vi "IMAQdx Acquisition Template (Host)withExtreme.vi"() -> ()   [LabVIEW 2016]
uses:
  <vilib>/userdefined/High Color/IMAQdx.ctl
  <vilib>/vision/driver/IMAQdx.llb/IMAQdx Acquisition Mode.ctl
  <vilib>/vision/driver/IMAQdx.llb/IMAQdx Buffer Number Mode.ctl
  <vilib>/FPGAPlugInAG/roboRIO/niLvFpga_Open_roboRIO.vi
  <vilib>/rvi/interface/common/dynamic/niFpgaDynamicAddResources.vi
  <vilib>/FPGAPlugInAG/Dynamic/niLvFpga_Download_Dynamic.vi
  <vilib>/FPGAPlugInAG/Dynamic/niLvFpga_Run_Dynamic.vi
  <vilib>/visionFPGA/Basics/Configure Image Transfer to Target/IMAQ FPGA Configure Image Transfer to Target U32.vi
  <vilib>/Utility/error.llb/Error Cluster From Error Code.vi
  <vilib>/rvi/errors/niLvFpgaAdjustHostInterfaceError.vi
  <vilib>/visionFPGA/Basics/Image Transfer to Target/IMAQ FPGA Image Transfer to Target U32.vi
  <vilib>/rvi/interface/common/niFpgaWaitOnOcc.vi
  <vilib>/FPGAPlugInAG/Dynamic/niLvFpga_Close_Dynamic.vi
  <vilib>/rvi/interface/nirviOpenFPGA/nirviOpenFPGA.xnode
  FPGA Bitfiles/ImageProcessingw_FPGATarget2_ImageProcessingw_ZcF2hsHpmf8.lvbitx
  <vilib>/rvi/interface/nirviMethod/nirviMethod.xnode
  <vilib>/rvi/interface/nirviReadWriteControl/nirviReadWriteControl.xnode
  <vilib>/rvi/interface/nirviCloseFPGA/nirviCloseFPGA.xnode
  <vilib>/vision/driver/NI_Vision_Acquisition_Software.lvlib
  <resource>/objmgr/imaqdx.rc
  <vilib>/visionFPGA/NI_VDM_FPGA_Basics.lvlib
  <vilib>/rvi/interface/Simulation/niFpgaSimulationCallBeginRW.vi
  <vilib>/rvi/errors/niLvFpgaMergeErrorWithErrorCode.vi
  <vilib>/FPGAPlugInAG/Dynamic/niLvFpga_ReadFifo_Dynamic.vi
  <vilib>/FPGAPlugInAG/Dynamic/niLvFpga_ConfigureFifo_Dynamic.vi
  <vilib>/FPGAPlugInAG/Dynamic/niLvFpga_StartFifo_Dynamic.vi
  NiFpgaLv.dll
panel:
  out "OriImage Err out":errorcluster
  out "Image":T1(plugin-control)
  out "Count":i32
  out "error out 2":errorcluster
  in  "Camera":T2
  out "Error Out":errorcluster
  in  "Stop":bool
  # "Overview: Demonstrates how to acquire an image from a camera using the IMAQdx API, transfer the image to a FPGA target for processing, and retrieve the processed image for display or further processing on the host.\nRequirements:\n- LabVIEW FPGA\n- Vision Acquisition Software\n- Vision Development Module\nInstructions:\n1. Select a Camera\n2. Run the VI."
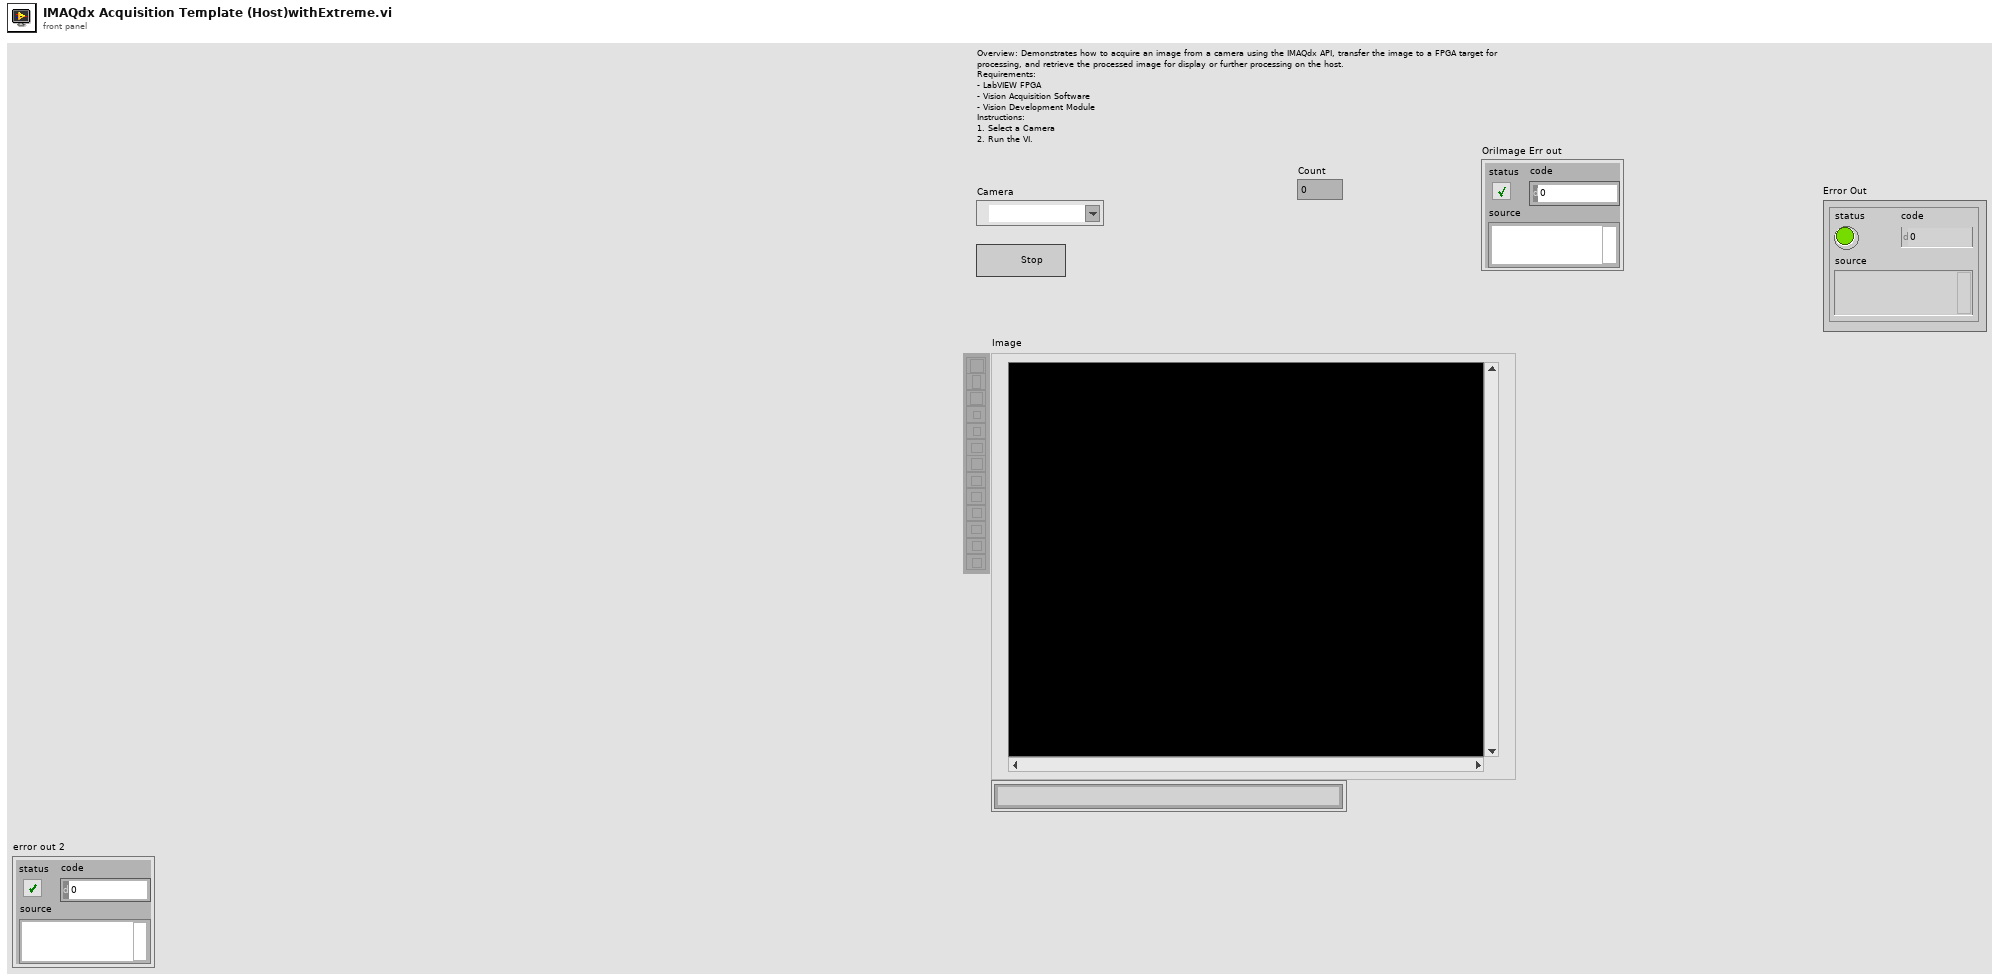
[diagram p1: front panel]
types:
  T1 = typedef "IMAQ Image.ctl" = refnum<image>
  T2 = typedef "IMAQdx.ctl" = refnum<k21>
  T3 = typedef "Image Type" = u32
  T4 = typedef "NI_Vision_Acquisition_Software.lvlib/IMAQdx Acquisition Mode.ctl" = enum32{"One Shot", "Continuous"}
  T5 = typedef "NI_Vision_Acquisition_Software.lvlib/IMAQdx Buffer Number Mode.ctl" = enum32{"Next", "Last", "Buffer Number", "Every", "Last New"}
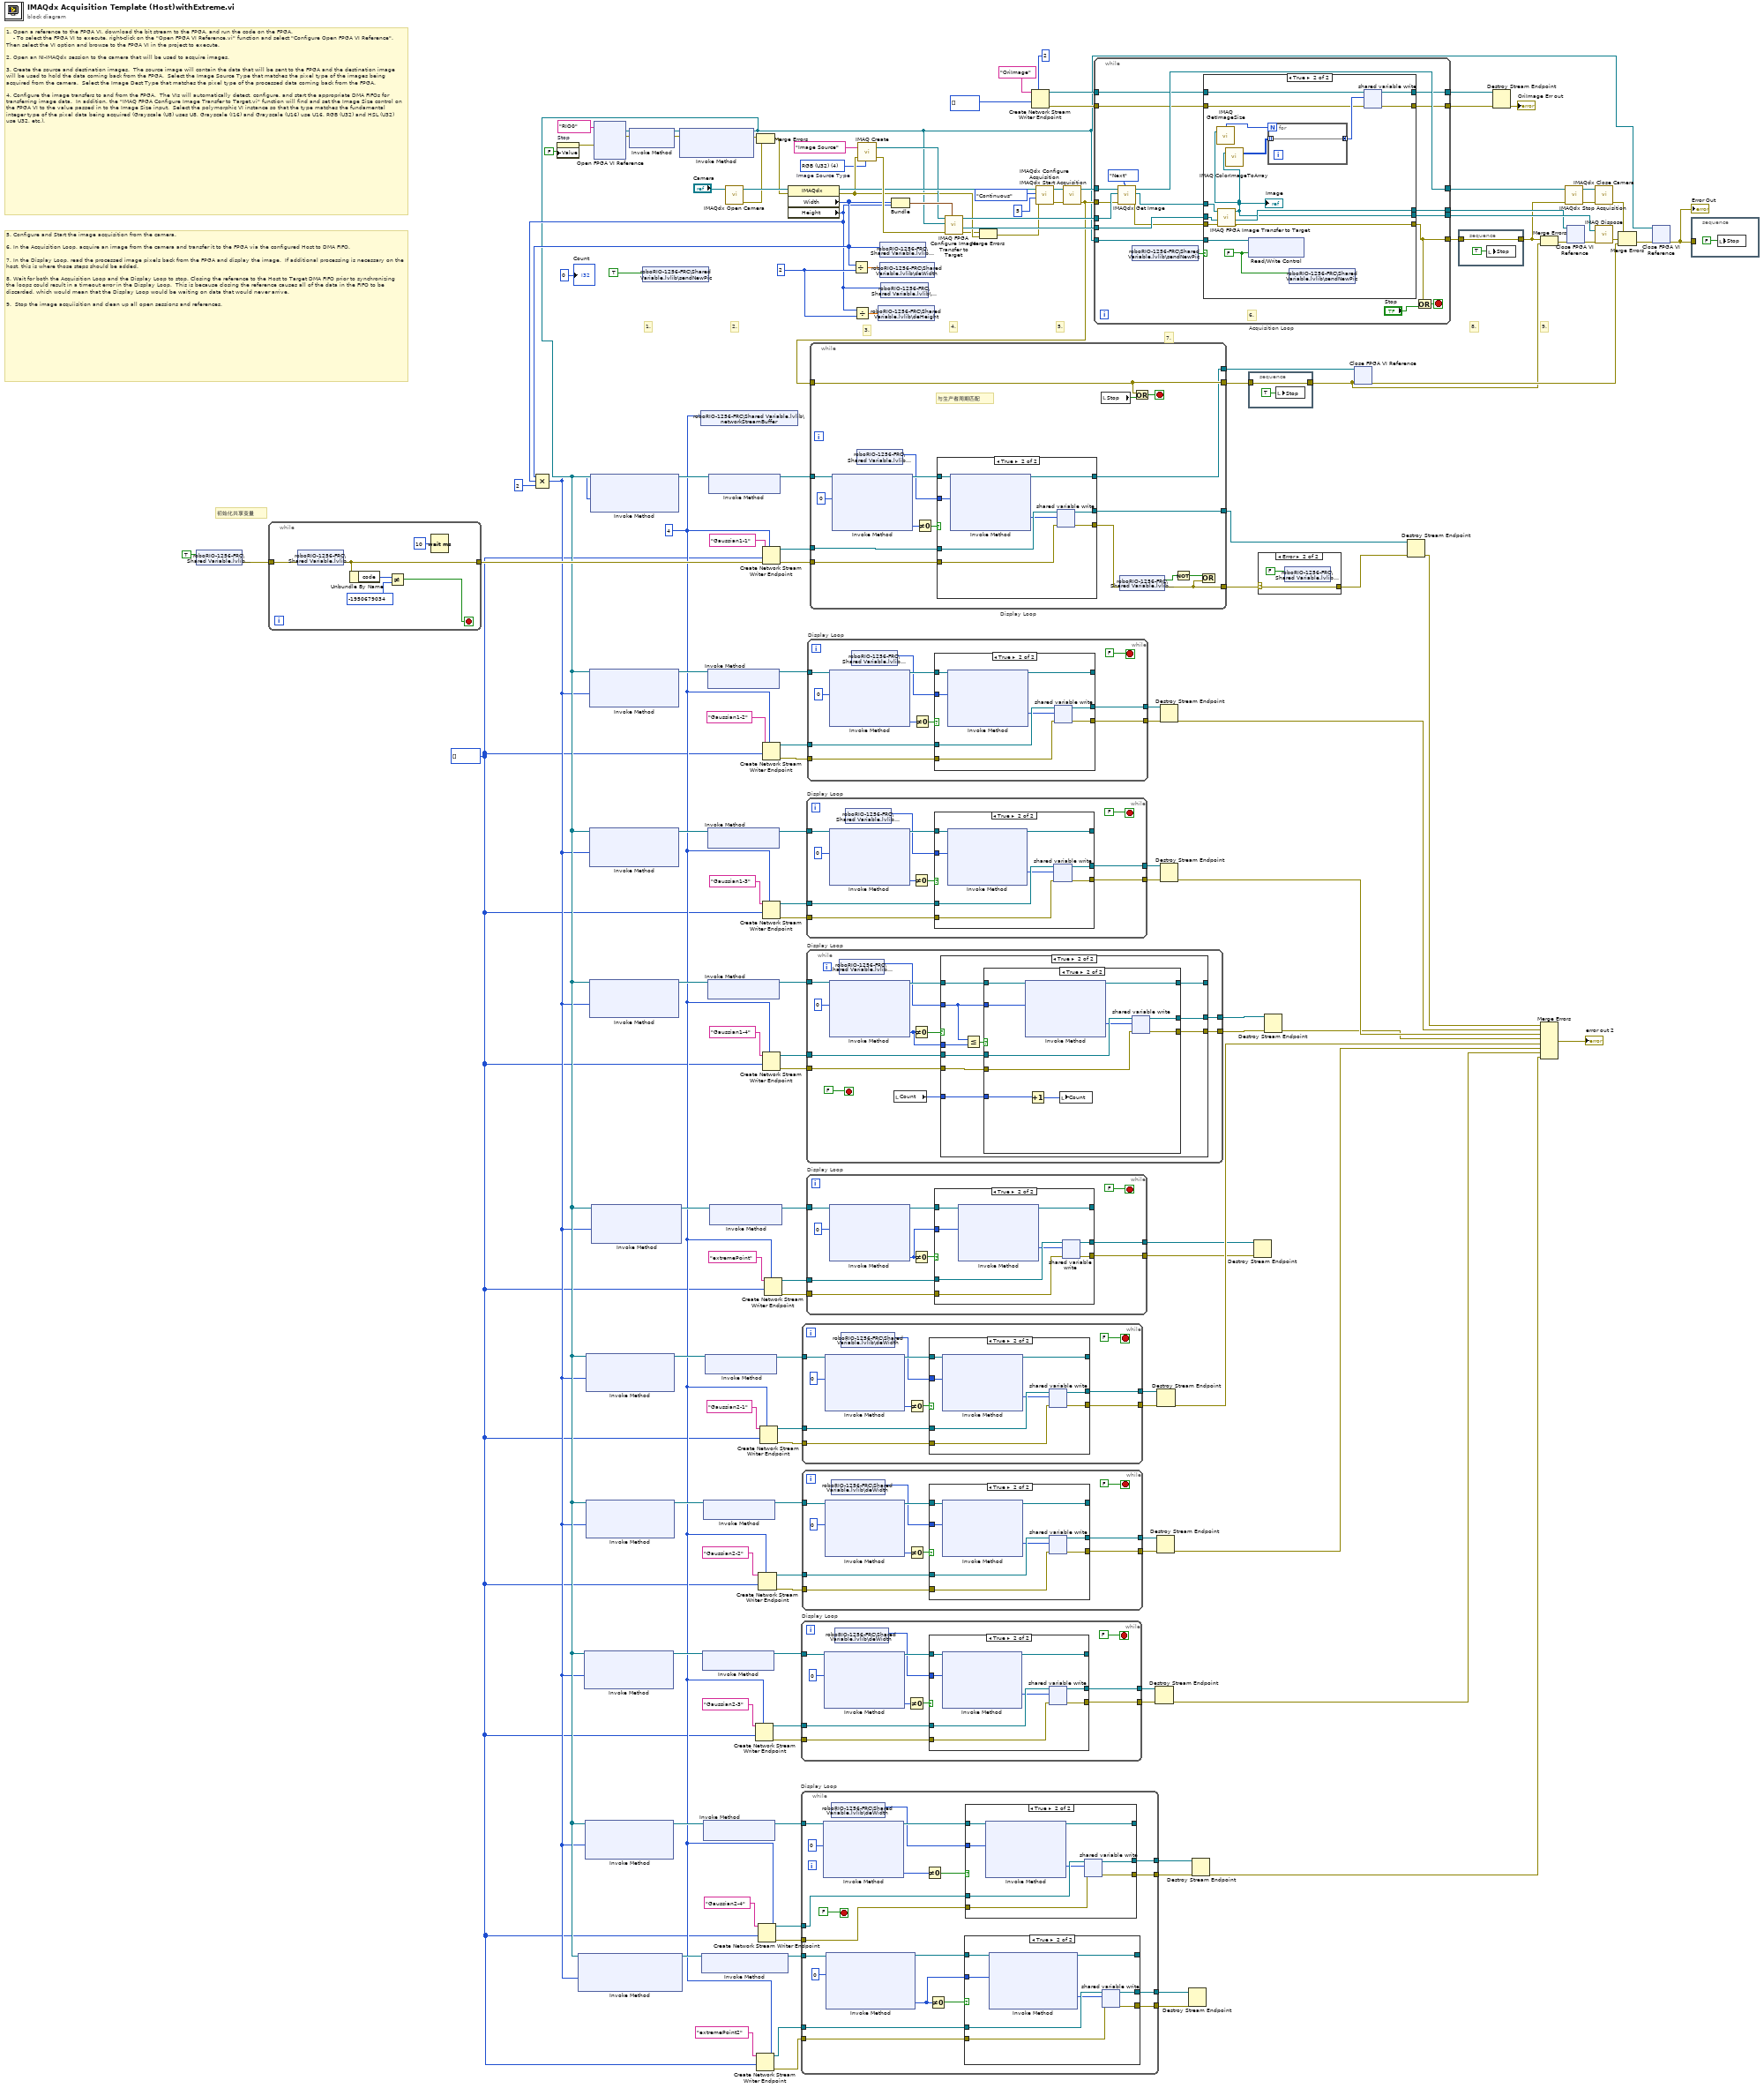
[diagram p0: block diagram]
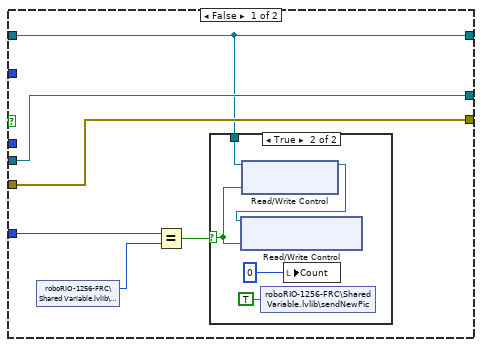
[diagram p6: hidden frame]
diagram:
  w21 = u32 2 ("y")
  w10 = i32[] []
  w12 = 4 ("writer buffer size")
  w112 = T3 4 items=["Grayscale (U8)", "Grayscale (I16)", "Grayscale (SGL)", "Complex (CSG)", "RGB (U32)", "HSL (U32)", "RGB (U64)", "Grayscale (U16)"]  # Image Source Type
  # "初始化共享变量"
  # "5. Configure and Start the image acquisition from the camera.\n\n6. In the Acquisition Loop, acquire an image from the camera and transfer it to the FPGA via the configured Host to DMA FIFO.\n\n7. In the Display Loop, read the processed image pixels back from the FPGA and display the image.  If additional processing is necessary on the host, this is where those steps should be added.\n\n8. Wait for both the Acquisition Loop and the Display Loop to stop. Closing the reference to the Host to Target DMA FIFO prior to synchronizing the loops could result in a timeout error in the Display Loop.  This is because closing the reference causes all of the data in the FIFO to be discarded, which would mean that the Display Loop would be waiting on data that would never arrive.\n\n9.  Stop the image acquiisition and clean up all open sessions and references."
  # "1. Open a reference to the FPGA VI, download the bit stream to the FPGA, and run the code on the FPGA.\n    - To select the FPGA VI to execute, right-click on the \"Open FPGA VI Reference.vi\" function and select \"Configure Open FPGA VI Reference\".  Then select the VI option and browse to the FPGA VI in the project to execute.\n\n2. Open an NI-IMAQdx session to the camera that will be used to acquire images.\n\n3. Create the source and destination images.  The source image will contain the data that will be sent to the FPGA and the destination image will be used to hold the data coming back from the FPGA.  Select the Image Source Type that matches the pixel type of the images being acquired from the camera.  Select the Image Dest Type that matches the pixel type of the processed data coming back from the FPGA.\n\n4. Configure the image transfers to and from the FPGA.  The VIs will automatically detect, configure, and start the appropriate DMA FIFOs for transferring image data.  In addition, the \"IMAQ FPGA Configure Image Transfer to Target.vi\" function will find and set the Image Size control on the FPGA VI to the value passed in to the Image Size input.  Select the polymorphic VI instance so that the type matches the fundamental integer type of the pixel data being acquired (Grayscale (U8) uses U8, Grayscale (I16) and Grayscale (U16) use U16, RGB (U32) and HSL (U32) use U32, etc.)."
  # "9."
  # "8."
  # "7."
  # "6."
  # "5."
  # "4."
  # "3."
  # "2."
  # "1."
  n1 = shared-variable "roboRIO-1256-FRC\\Shared Variable.lvlib\\Active"(TRUE ("Active?")) -> (error out=w98:errorcluster)  [unwired: 1 in]
  n2 = while {
    tunnel: w98 -> [w155]
    tunnel: [w152] -> w97
    stop <- w151 stop-if-true
    n3 = shared-variable "roboRIO-1256-FRC\\Shared Variable.lvlib\\Active"(error in=w155) -> (error out=w152:errorcluster)  [unwired: 1 out]
    n4 = Unbundle By Name(w152) -> ("code"=w154:i32)
    n5 = Not Equal?(x=w154, y=-1950679034) -> (x != y?=w151:bool)
    n6 = Wait (ms)(milliseconds to wait=u32 10) -> ()  [unwired: 1 out]
  }
  n7 = property on="Stop" class="Bool (strict)"("Value"=FALSE ("Stop")) -> (error out=w147:errorcluster)  [unwired: 2 in, 1 out]
  n8 = xnode "Open FPGA VI Reference"("error in"=w147, "resource name"=tag "RIO0") -> ("FPGA VI Reference Out"=w143:refnum<k20>, "error out"=w144:errorcluster)
  n9 = xnode "Invoke Method"("FPGA VI Reference In"=w143, "error in"=w144) -> ("FPGA VI Reference Out"=w146:refnum<k20>, "error out"=w145:errorcluster)
  n10 = shared-variable "roboRIO-1256-FRC\\Shared Variable.lvlib\\sendNewPic"(TRUE) -> ()  [unwired: 1 in, 1 out]
  n11 = xnode "Invoke Method"("FPGA VI Reference In"=w146, "error in"=w145) -> ("FPGA VI Reference Out"=w14:refnum<k20>, "error out"=w132:errorcluster)  [unwired: 1 in]
  n12 = shared-variable "roboRIO-1256-FRC\\Shared Variable.lvlib\\networkStreamBuffer"(w12) -> ()  [unwired: 1 in, 1 out]
  n13 = call <vilib>:"IMAQdx Open Camera.vi"("Session In"="Camera") -> ("error out"=w117:errorcluster, "Session Out"=w118:T2)  [unwired: 9 in]
  n14 = Create Network Stream Writer Endpoint(7:w12, 9:w10, 11:"Gaussian2-3" ("writer name")) -> (0:w34:errorcluster, 3:w33:refnum<k21>)  [unwired: 4 in]
  n15 = Create Network Stream Writer Endpoint(7:w12, 9:w10, 11:"extremePoint2" ("writer name")) -> (0:w8:errorcluster, 3:w9:refnum<k21>)  [unwired: 4 in]
  n16 = Merge Errors(w132, w117) -> (w116:errorcluster)
  n17 = Create Network Stream Writer Endpoint(7:w12, 9:w10, 11:"Gaussian2-4" ("writer name")) -> (0:w59:errorcluster, 3:w60:refnum<k21>)  [unwired: 4 in]
  n18 = Create Network Stream Writer Endpoint(7:w12, 9:w10, 11:"Gaussian2-2" ("writer name")) -> (0:w41:errorcluster, 3:w42:refnum<k21>)  [unwired: 4 in]
  n19 = Create Network Stream Writer Endpoint(7:w12, 9:w10, 11:"Gaussian2-1" ("writer name")) -> (0:w48:errorcluster, 3:w47:refnum<k21>)  [unwired: 4 in]
  n20 = Create Network Stream Writer Endpoint(7:w12, 8:w97, 9:w10, 11:"Gaussian1-1" ("writer name")) -> (0:w93:errorcluster, 3:w92:refnum<k21>)  [unwired: 3 in]
  n21 = Create Network Stream Writer Endpoint(7:w12, 9:w10, 11:"Gaussian1-2" ("writer name")) -> (0:w74:errorcluster, 3:w75:refnum<k21>)  [unwired: 4 in]
  n22 = Create Network Stream Writer Endpoint(7:w12, 9:w10, 11:"Gaussian1-3" ("writer name")) -> (0:w69:errorcluster, 3:w68:refnum<k21>)  [unwired: 4 in]
  n23 = Create Network Stream Writer Endpoint(7:w12, 9:w10, 11:"Gaussian1-4" ("writer name")) -> (0:w53:errorcluster, 3:w54:refnum<k21>)  [unwired: 4 in]
  n24 = Create Network Stream Writer Endpoint(7:w12, 9:w10, 11:"extremePoint" ("writer name")) -> (0:w3:errorcluster, 3:w4:refnum<k21>)  [unwired: 4 in]
  n25 = property class="IMAQdx"(reference=w118, error in=w116) -> (reference out=w125:T2, error out=w113:errorcluster, "Width"=w23:u32, "Height"=w20:u32)
  n26 = Compound Arithmetic op=MULTIPLY(w23, w20, u32 2 ("value")) -> (w13:u32)
  n27 = xnode "Invoke Method"("FPGA VI Reference In"=w14, "Requested Depth"=w13) -> ("FPGA VI Reference Out"=w16:refnum<k20>)  [unwired: 1 in, 2 out]
  n28 = xnode "Invoke Method"("FPGA VI Reference In"=w14, "Requested Depth"=w13) -> ("FPGA VI Reference Out"=w35:refnum<k20>)  [unwired: 1 in, 2 out]
  n29 = xnode "Invoke Method"("FPGA VI Reference In"=w14, "Requested Depth"=w13) -> ("FPGA VI Reference Out"=w58:refnum<k20>)  [unwired: 1 in, 2 out]
  n30 = xnode "Invoke Method"("FPGA VI Reference In"=w14, "Requested Depth"=w13) -> ("FPGA VI Reference Out"=w30:refnum<k20>)  [unwired: 1 in, 2 out]
  n31 = xnode "Invoke Method"("FPGA VI Reference In"=w14, "Requested Depth"=w13) -> ("FPGA VI Reference Out"=w40:refnum<k20>)  [unwired: 1 in, 2 out]
  n32 = xnode "Invoke Method"("FPGA VI Reference In"=w14, "Requested Depth"=w13) -> ("FPGA VI Reference Out"=w73:refnum<k20>)  [unwired: 1 in, 2 out]
  n33 = xnode "Invoke Method"("FPGA VI Reference In"=w14, "Requested Depth"=w13) -> ("FPGA VI Reference Out"=w70:refnum<k20>)  [unwired: 1 in, 2 out]
  n34 = xnode "Invoke Method"("FPGA VI Reference In"=w14, "Requested Depth"=w13) -> ("FPGA VI Reference Out"=w52:refnum<k20>)  [unwired: 1 in, 2 out]
  n35 = xnode "Invoke Method"("FPGA VI Reference In"=w14, "Requested Depth"=w13) -> ("FPGA VI Reference Out"=w102:refnum<k20>)  [unwired: 1 in, 2 out]
  n36 = xnode "Invoke Method"("FPGA VI Reference In"=w14, "Requested Depth"=w13) -> ("FPGA VI Reference Out"=w17:refnum<k20>)  [unwired: 1 in, 2 out]
  n37 = xnode "Invoke Method"("FPGA VI Reference In"=w16) -> ("FPGA VI Reference Out"=w11:refnum<k20>)  [unwired: 1 in, 1 out]
  n38 = xnode "Invoke Method"("FPGA VI Reference In"=w35) -> ("FPGA VI Reference Out"=w36:refnum<k20>)  [unwired: 1 in, 1 out]
  n39 = xnode "Invoke Method"("FPGA VI Reference In"=w58) -> ("FPGA VI Reference Out"=w57:refnum<k20>)  [unwired: 1 in, 1 out]
  n40 = xnode "Invoke Method"("FPGA VI Reference In"=w40) -> ("FPGA VI Reference Out"=w39:refnum<k20>)  [unwired: 1 in, 1 out]
  n41 = xnode "Invoke Method"("FPGA VI Reference In"=w30) -> ("FPGA VI Reference Out"=w29:refnum<k20>)  [unwired: 1 in, 1 out]
  n42 = xnode "Invoke Method"("FPGA VI Reference In"=w73) -> ("FPGA VI Reference Out"=w72:refnum<k20>)  [unwired: 1 in, 1 out]
  n43 = xnode "Invoke Method"("FPGA VI Reference In"=w70) -> ("FPGA VI Reference Out"=w71:refnum<k20>)  [unwired: 1 in, 1 out]
  n44 = xnode "Invoke Method"("FPGA VI Reference In"=w52) -> ("FPGA VI Reference Out"=w51:refnum<k20>)  [unwired: 1 in, 1 out]
  n45 = xnode "Invoke Method"("FPGA VI Reference In"=w102) -> ("FPGA VI Reference Out"=w101:refnum<k20>)  [unwired: 1 in, 1 out]
  n46 = xnode "Invoke Method"("FPGA VI Reference In"=w17) -> ("FPGA VI Reference Out"=w5:refnum<k20>)  [unwired: 1 in, 1 out]
  n47 = while "Display Loop" {
    tunnel: [w175] -> w63
    tunnel: w59 -> [w174]
    tunnel: w60 -> [w173]
    tunnel: [w168] -> w62
    tunnel: w57 -> [w167]
    tunnel: w11 -> [w161]
    tunnel: w9 -> [w160]
    tunnel: w8 -> [w159]
    tunnel: [w158] -> w7
    tunnel: [w157] -> w6
    stop <- FALSE stop-if-true
    n48 = xnode "Invoke Method"("FPGA VI Reference In"=w167, "Number of Elements"=u32 0) -> ("FPGA VI Reference Out"=w170:refnum<k20>, "Elements Remaining"=w165:u32)  [unwired: 2 in, 2 out]
    n49 = xnode "Invoke Method"("FPGA VI Reference In"=w161, "Number of Elements"=u32 0) -> ("FPGA VI Reference Out"=w164:refnum<k20>, "Elements Remaining"=w156:u32)  [unwired: 2 in, 2 out]
    n50 = shared-variable "roboRIO-1256-FRC\\Shared Variable.lvlib\\deWidth"() -> (w166:u16)  [unwired: 1 in, 1 out]
    n51 = Not Equal To 0?(x=w165) -> (x != 0?=w172:bool)
    n52 = Not Equal To 0?(x=w156) -> (x != 0?=w162:bool)
    n53 = case shown="True" w162 {
      tunnel: w164 -> [w176 w186]
      tunnel: [w178 w185] -> w158
      tunnel: w159 -> [w177 w184]
      tunnel: w160 -> [w178 w183]
      tunnel: [w177 w182] -> w157
      tunnel: [w176 w181] -> _
      tunnel: w156 -> [_ w179]
      frame False {
      }
      frame True {
        n54 = xnode "Invoke Method"("FPGA VI Reference In"=w186, "Number of Elements"=w179) -> ("FPGA VI Reference Out"=w181:refnum<k20>, "Data"=w180:u16[])  [unwired: 2 in, 2 out]
        n55 = shared-variable-write(w183, w184, w180) -> (w185:refnum<k21>, w182:errorcluster)  [unwired: 1 in, 1 out]
      }
    }
    n56 = case shown="True" w172 {
      tunnel: w170 -> [w187 w197]
      tunnel: [w189 w196] -> w175
      tunnel: w174 -> [w188 w195]
      tunnel: w173 -> [w189 w194]
      tunnel: [w188 w193] -> w168
      tunnel: [w187 w192] -> _
      tunnel: w166 -> [_ w191]
      frame False {
      }
      frame True {
        n57 = xnode "Invoke Method"("FPGA VI Reference In"=w197, "Number of Elements"=w191) -> ("FPGA VI Reference Out"=w192:refnum<k20>, "Data"=w190:u8[])  [unwired: 2 in, 2 out]
        n58 = shared-variable-write(w194, w195, w190) -> (w196:refnum<k21>, w193:errorcluster)  [unwired: 1 in, 1 out]
      }
    }
  }
  n59 = while "Display Loop" {
    tunnel: [w208] -> w31
    tunnel: w34 -> [w207]
    tunnel: w33 -> [w206]
    tunnel: [w200] -> w32
    tunnel: w36 -> [w199]
    stop <- FALSE stop-if-true
    (unwired) u32 640 ("Number of Elements")
    n60 = xnode "Invoke Method"("FPGA VI Reference In"=w199, "Number of Elements"=u32 0) -> ("FPGA VI Reference Out"=w202:refnum<k20>, "Elements Remaining"=w203:u32)  [unwired: 2 in, 2 out]
    n61 = shared-variable "roboRIO-1256-FRC\\Shared Variable.lvlib\\deWidth"() -> (w198:u16)  [unwired: 1 in, 1 out]
    n62 = Not Equal To 0?(x=w203) -> (x != 0?=w205:bool)
    n63 = case shown="True" w205 {
      tunnel: w202 -> [w209 w219]
      tunnel: [w211 w218] -> w208
      tunnel: w207 -> [w210 w217]
      tunnel: w206 -> [w211 w216]
      tunnel: [w210 w215] -> w200
      tunnel: [w209 w213] -> _
      tunnel: w198 -> [_ w212]
      frame False {
      }
      frame True {
        n64 = xnode "Invoke Method"("FPGA VI Reference In"=w219, "Number of Elements"=w212) -> ("FPGA VI Reference Out"=w213:refnum<k20>, "Data"=w214:u8[])  [unwired: 2 in, 2 out]
        n65 = shared-variable-write(w216, w217, w214) -> (w218:refnum<k21>, w215:errorcluster)  [unwired: 1 in, 1 out]
      }
    }
  }
  n66 = while "Display Loop" {
    tunnel: [w230] -> w45
    tunnel: w48 -> [w229]
    tunnel: w47 -> [w228]
    tunnel: [w222] -> w46
    tunnel: w29 -> [w221]
    stop <- FALSE stop-if-true
    (unwired) u32 640 ("Number of Elements")
    n67 = xnode "Invoke Method"("FPGA VI Reference In"=w221, "Number of Elements"=u32 0) -> ("FPGA VI Reference Out"=w224:refnum<k20>, "Elements Remaining"=w225:u32)  [unwired: 2 in, 2 out]
    n68 = shared-variable "roboRIO-1256-FRC\\Shared Variable.lvlib\\deWidth"() -> (w220:u16)  [unwired: 1 in, 1 out]
    n69 = Not Equal To 0?(x=w225) -> (x != 0?=w227:bool)
    n70 = case shown="True" w227 {
      tunnel: w224 -> [w231 w241]
      tunnel: [w233 w240] -> w230
      tunnel: w229 -> [w232 w239]
      tunnel: w228 -> [w233 w238]
      tunnel: [w232 w237] -> w222
      tunnel: [w231 w235] -> _
      tunnel: w220 -> [_ w234]
      frame False {
      }
      frame True {
        n71 = xnode "Invoke Method"("FPGA VI Reference In"=w241, "Number of Elements"=w234) -> ("FPGA VI Reference Out"=w235:refnum<k20>, "Data"=w236:u8[])  [unwired: 2 in, 2 out]
        n72 = shared-variable-write(w238, w239, w236) -> (w240:refnum<k21>, w237:errorcluster)  [unwired: 1 in, 1 out]
      }
    }
  }
  n73 = while "Display Loop" {
    tunnel: [w252] -> w44
    tunnel: w41 -> [w251]
    tunnel: w42 -> [w250]
    tunnel: [w244] -> w43
    tunnel: w39 -> [w243]
    stop <- FALSE stop-if-true
    (unwired) u32 640 ("Number of Elements")
    n74 = xnode "Invoke Method"("FPGA VI Reference In"=w243, "Number of Elements"=u32 0) -> ("FPGA VI Reference Out"=w246:refnum<k20>, "Elements Remaining"=w247:u32)  [unwired: 2 in, 2 out]
    n75 = shared-variable "roboRIO-1256-FRC\\Shared Variable.lvlib\\deWidth"() -> (w242:u16)  [unwired: 1 in, 1 out]
    n76 = Not Equal To 0?(x=w247) -> (x != 0?=w249:bool)
    n77 = case shown="True" w249 {
      tunnel: w246 -> [w253 w263]
      tunnel: [w255 w262] -> w252
      tunnel: w251 -> [w254 w261]
      tunnel: w250 -> [w255 w260]
      tunnel: [w254 w259] -> w244
      tunnel: [w253 w257] -> _
      tunnel: w242 -> [_ w256]
      frame False {
      }
      frame True {
        n78 = xnode "Invoke Method"("FPGA VI Reference In"=w263, "Number of Elements"=w256) -> ("FPGA VI Reference Out"=w257:refnum<k20>, "Data"=w258:u8[])  [unwired: 2 in, 2 out]
        n79 = shared-variable-write(w260, w261, w258) -> (w262:refnum<k21>, w259:errorcluster)  [unwired: 1 in, 1 out]
      }
    }
  }
  n80 = while "Display Loop" {
    tunnel: [w274] -> w65
    tunnel: w69 -> [w273]
    tunnel: w68 -> [w272]
    tunnel: [w266] -> w66
    tunnel: w71 -> [w265]
    stop <- FALSE stop-if-true
    (unwired) u32 640 ("Number of Elements")
    n81 = xnode "Invoke Method"("FPGA VI Reference In"=w265, "Number of Elements"=u32 0) -> ("FPGA VI Reference Out"=w268:refnum<k20>, "Elements Remaining"=w269:u32)  [unwired: 2 in, 2 out]
    n82 = shared-variable "roboRIO-1256-FRC\\Shared Variable.lvlib\\Width"() -> (w264:u16)  [unwired: 1 in, 1 out]
    n83 = Not Equal To 0?(x=w269) -> (x != 0?=w271:bool)
    n84 = case shown="True" w271 {
      tunnel: w268 -> [w275 w285]
      tunnel: [w277 w284] -> w274
      tunnel: w273 -> [w276 w283]
      tunnel: w272 -> [w277 w282]
      tunnel: [w276 w281] -> w266
      tunnel: [w275 w279] -> _
      tunnel: w264 -> [_ w278]
      frame False {
      }
      frame True {
        n85 = xnode "Invoke Method"("FPGA VI Reference In"=w285, "Number of Elements"=w278) -> ("FPGA VI Reference Out"=w279:refnum<k20>, "Data"=w280:u8[])  [unwired: 2 in, 2 out]
        n86 = shared-variable-write(w282, w283, w280) -> (w284:refnum<k21>, w281:errorcluster)  [unwired: 1 in, 1 out]
      }
    }
  }
  n87 = while "Display Loop" {
    tunnel: [w297] -> w56
    tunnel: w53 -> [w296]
    tunnel: w54 -> [w295]
    tunnel: [w290] -> w55
    tunnel: w51 -> [w289]
    stop <- FALSE stop-if-true
    n88 = xnode "Invoke Method"("FPGA VI Reference In"=w289, "Number of Elements"=u32 0) -> ("FPGA VI Reference Out"=w292:refnum<k20>, "Elements Remaining"=w286:u32)  [unwired: 2 in, 2 out]
    n89 = shared-variable "roboRIO-1256-FRC\\Shared Variable.lvlib\\Width"() -> (w288:u16)  [unwired: 1 in, 1 out]
    n90 = local read "Count"() -> (w287:i32)
    n91 = Not Equal To 0?(x=w286) -> (x != 0?=w294:bool)
    n92 = case shown="True" w294 {
      tunnel: w292 -> [w298 w318]
      tunnel: [w303 w317] -> w297
      tunnel: w296 -> [w302 w316]
      tunnel: w295 -> [w303 w315]
      tunnel: [w302 w314] -> w290
      tunnel: [w298 w313] -> _
      tunnel: w288 -> [_ w310]
      tunnel: w287 -> [w300 w312]
      tunnel: w286 -> [_ w309]
      frame False {
        n93 = shared-variable "roboRIO-1256-FRC\\Shared Variable.lvlib\\Height"() -> (w299:u16)  [unwired: 1 in, 1 out]
        n94 = Equal?(x=w300, y=w299) -> (x = y?=w301:bool)
        n95 = case shown="True" w301 {
          selector: w301 -> [_ w305]
          tunnel: w298 -> [_ w308]
          frame False {
          }
          frame True {
            n96 = xnode "Read/Write Control"("FPGA VI Reference In"=w308, "StartOfImage"=w305) -> ("FPGA VI Reference Out"=w307:refnum<k20>)  [unwired: 1 in, 1 out]
            n97 = xnode "Read/Write Control"("FPGA VI Reference In"=w307, "Ready For Output"=w305) -> ()  [unwired: 1 in, 2 out]
            n98 = shared-variable "roboRIO-1256-FRC\\Shared Variable.lvlib\\sendNewPic"(TRUE ("start")) -> ()  [unwired: 1 in, 1 out]
            n99 = local write "Count"(0) -> ()
          }
        }
      }
      frame True {
        n100 = Less Or Equal?(x=w310, y=w309) -> (x <= y?=w311:bool)
        n101 = case shown="True" w311 {
          tunnel: w318 -> [w321 w331]
          tunnel: [w320 w330] -> w317
          tunnel: w316 -> [w319 w329]
          tunnel: w315 -> [w320 w328]
          tunnel: [w319 w327] -> w314
          tunnel: [w321 w325] -> w313
          tunnel: w310 -> [_ w324]
          tunnel: w312 -> [_ w323]
          frame False {
          }
          frame True {
            n102 = xnode "Invoke Method"("FPGA VI Reference In"=w331, "Number of Elements"=w324) -> ("FPGA VI Reference Out"=w325:refnum<k20>, "Data"=w326:u8[])  [unwired: 2 in, 2 out]
            n103 = Increment(x=w323) -> (x+1=w322:i32)
            n104 = local write "Count"(w322) -> ()
            n105 = shared-variable-write(w328, w329, w326) -> (w330:refnum<k21>, w327:errorcluster)  [unwired: 1 in, 1 out]
          }
        }
      }
    }
  }
  n106 = while "Display Loop" {
    tunnel: [w341] -> w2
    tunnel: [w336] -> w1
    tunnel: w5 -> [w335]
    tunnel: w4 -> [w334]
    tunnel: w3 -> [w333]
    stop <- FALSE stop-if-true
    (unwired) u32 640 ("Number of Elements")
    n107 = xnode "Invoke Method"("FPGA VI Reference In"=w335, "Number of Elements"=u32 0) -> ("FPGA VI Reference Out"=w338:refnum<k20>, "Elements Remaining"=w332:u32)  [unwired: 2 in, 2 out]
    n108 = Not Equal To 0?(x=w332) -> (x != 0?=w340:bool)
    n109 = case shown="True" w340 {
      tunnel: w338 -> [w342 w352]
      tunnel: [w344 w351] -> w341
      tunnel: w333 -> [w343 w350]
      tunnel: w334 -> [w344 w349]
      tunnel: [w343 w348] -> w336
      tunnel: [w342 w346] -> _
      tunnel: w332 -> [_ w345]
      frame False {
      }
      frame True {
        n110 = xnode "Invoke Method"("FPGA VI Reference In"=w352, "Number of Elements"=w345) -> ("FPGA VI Reference Out"=w346:refnum<k20>, "Data"=w347:u16[])  [unwired: 2 in, 2 out]
        n111 = shared-variable-write(w349, w350, w347) -> (w351:refnum<k21>, w348:errorcluster)  [unwired: 1 in, 1 out]
      }
    }
  }
  n112 = while "Display Loop" {
    tunnel: [w363] -> w82
    tunnel: w74 -> [w362]
    tunnel: w75 -> [w361]
    tunnel: [w355] -> w81
    tunnel: w72 -> [w354]
    stop <- FALSE stop-if-true
    (unwired) u32 640 ("Number of Elements")
    n113 = xnode "Invoke Method"("FPGA VI Reference In"=w354, "Number of Elements"=u32 0) -> ("FPGA VI Reference Out"=w357:refnum<k20>, "Elements Remaining"=w358:u32)  [unwired: 2 in, 2 out]
    n114 = shared-variable "roboRIO-1256-FRC\\Shared Variable.lvlib\\Width"() -> (w353:u16)  [unwired: 1 in, 1 out]
    n115 = Not Equal To 0?(x=w358) -> (x != 0?=w360:bool)
    n116 = case shown="True" w360 {
      tunnel: w357 -> [w364 w374]
      tunnel: [w366 w373] -> w363
      tunnel: w362 -> [w365 w372]
      tunnel: w361 -> [w366 w371]
      tunnel: [w365 w370] -> w355
      tunnel: [w364 w368] -> _
      tunnel: w353 -> [_ w367]
      frame False {
      }
      frame True {
        n117 = xnode "Invoke Method"("FPGA VI Reference In"=w374, "Number of Elements"=w367) -> ("FPGA VI Reference Out"=w368:refnum<k20>, "Data"=w369:u8[])  [unwired: 2 in, 2 out]
        n118 = shared-variable-write(w371, w372, w369) -> (w373:refnum<k21>, w370:errorcluster)  [unwired: 1 in, 1 out]
      }
    }
  }
  n119 = Divide(x=w23, y=w21) -> (x/y=w22:dbl)
  n120 = Divide(x=w20, y=w21) -> (x/y=w19:dbl)
  n121 = call "IMAQ Create"("Image Name"="Image Source", "Image Type"=w112, "error in (no error)"=w113) -> ("New Image"=w123:T1, "error out"=w131:errorcluster)  [unwired: 2 in]
  n122 = shared-variable "roboRIO-1256-FRC\\Shared Variable.lvlib\\deHeight"(w19) -> ()  [unwired: 1 in, 1 out]
  n123 = shared-variable "roboRIO-1256-FRC\\Shared Variable.lvlib\\Width"(w23) -> ()  [unwired: 1 in, 1 out]
  n124 = shared-variable "roboRIO-1256-FRC\\Shared Variable.lvlib\\deWidth"(w22) -> ()  [unwired: 1 in, 1 out]
  n125 = shared-variable "roboRIO-1256-FRC\\Shared Variable.lvlib\\Height"(w20) -> ()  [unwired: 1 in, 1 out]
  n126 = Bundle("Width"=w23, "Height"=w20) -> (w130:cluster{"Width":u32, "Height":u32})  [unwired: 1 in]
  n127 = call-poly <vilib>:"IMAQ FPGA Configure Image Transfer to Target.vi"("Image Size"=w130, "error in (no error)"=w131, "FPGA VI Reference In"=w14, "Image"=w123) -> ("error out"=w106:errorcluster, "DMA FIFO Reference Out"=w141:refnum<k20>, "Image Out"=w142:T1)  [unwired: 4 in, 1 out]
  n128 = Merge Errors(w106, w113) -> (w105:errorcluster)
  n129 = Create Network Stream Writer Endpoint(7:2 ("writer buffer size"), 9:i32[] [], 11:"OriImage" ("writer name")) -> (0:w86:errorcluster, 3:w87:refnum<k21>)  [unwired: 4 in]
  n130 = call <vilib>:"IMAQdx Configure Acquisition.vi"("error in"=w105, "Number of Buffers"=u32 5, "Continuous?"=IMAQdx_Acquisition_Mode."Continuous", "Session In"=w125) -> ("error out"=w128:errorcluster, "Session Out"=w129:T2)  [unwired: 6 in]
  n131 = call <vilib>:"IMAQdx Start Acquisition.vi"("error in"=w128, "Session In"=w129) -> ("error out"=w104:errorcluster, "Session Out"=w124:T2)  [unwired: 8 in]
  n132 = while "Display Loop" {
    tunnel: w104 -> [w390]
    tunnel: [w378] -> w138
    tunnel: [w390] -> w137
    tunnel: w101 -> [w379]
    tunnel: [w388] -> w95
    tunnel: [w387] -> w94
    tunnel: w93 -> [w386]
    tunnel: w92 -> [w385]
    stop <- w391 stop-if-true
    (unwired) u32 640 ("Number of Elements")
    # "与生产者周期匹配"
    n133 = xnode "Invoke Method"("FPGA VI Reference In"=w379, "Number of Elements"=u32 0) -> ("FPGA VI Reference Out"=w376:refnum<k20>, "Elements Remaining"=w377:u32)  [unwired: 2 in, 2 out]
    n134 = shared-variable "roboRIO-1256-FRC\\Shared Variable.lvlib\\Width"() -> (w375:u16)  [unwired: 1 in, 1 out]
    n135 = Not Equal To 0?(x=w377) -> (x != 0?=w381:bool)
    n136 = case shown="True" w381 {
      tunnel: w376 -> [w392 w402]
      tunnel: [w394 w401] -> w387
      tunnel: w386 -> [w393 w400]
      tunnel: w385 -> [w394 w399]
      tunnel: [w393 w398] -> w384
      tunnel: [w392 w396] -> w378
      tunnel: w375 -> [_ w395]
      frame False {
      }
      frame True {
        n137 = xnode "Invoke Method"("FPGA VI Reference In"=w402, "Number of Elements"=w395) -> ("FPGA VI Reference Out"=w396:refnum<k20>, "Data"=w397:u8[])  [unwired: 2 in, 2 out]
        n138 = shared-variable-write(w399, w400, w397) -> (w401:refnum<k21>, w398:errorcluster)  [unwired: 1 in, 1 out]
      }
    }
    n139 = local read "Stop"() -> (w389:bool)
    n140 = shared-variable "roboRIO-1256-FRC\\Shared Variable.lvlib\\Active"(error in=w384) -> (w382:bool, error out=w388:errorcluster)
    n141 = Or(x=w390, y=w389) -> (x .or. y?=w391:bool)
    n142 = Not(x=w382) -> (.not. x?=w383:bool)
    n143 = Or(x=w383, y=w388) -> ()  [unwired: 1 out]
  }
  n144 = while "Acquisition Loop" {
    tunnel: [w412] -> w110
    tunnel: w142 -> [w417]
    tunnel: w141 -> [w414]
    tunnel: [w413] -> w111
    tunnel: [w410] -> w140
    tunnel: w124 -> [w418]
    tunnel: [w416] -> w120
    tunnel: w104 -> [w415]
    tunnel: w14 -> [w408]
    tunnel: w87 -> [w407]
    tunnel: w86 -> [w406]
    tunnel: [w405] -> w85
    tunnel: [w404] -> w84
    stop <- w420 stop-if-true
    n145 = call <vilib>:"IMAQdx Get Image.vi"("Buffer Number Mode (Next)"=IMAQdx_Buffer_Number_Mode."Next", "error in"=w415, "Image In"=w417, "Session In"=w418) -> ("error out"=w409:errorcluster, "Image Out"=w411:T1, "Session Out"=w416:T2)  [unwired: 4 in, 1 out]
    n146 = shared-variable "roboRIO-1256-FRC\\Shared Variable.lvlib\\sendNewPic"() -> (w403:bool)  [unwired: 1 in, 1 out]
    n147 = case shown="True" w403 {
      tunnel: w414 -> [w426 w441]
      tunnel: [w426 w437] -> w413
      tunnel: [w425 w438] -> w412
      tunnel: w411 -> [w424 w440]
      tunnel: [w424 w432] -> w410
      tunnel: w409 -> [w425 w439]
      tunnel: w408 -> [_ w435]
      tunnel: w407 -> [w423 w430]
      tunnel: w406 -> [w422 w429]
      tunnel: [w423 w428] -> w405
      tunnel: [w422 w427] -> w404
      frame False {
      }
      frame True {
        w436 = FALSE ("EndOfImage")
        n148 = call-poly <vilib>:"IMAQ FPGA Image Transfer to Target.vi"("error in (no error)"=w439, "DMA FIFO Reference In"=w441, "Image"=w440) -> ("error out"=w438:errorcluster, "DMA FIFO Reference Out"=w437:refnum<k20>, "Image Out"=w432:T1)  [unwired: 6 in]
        "Image" <- w432
        n149 = call "IMAQ GetImageSize"("Image"=w432) -> ("X Resolution"=w434:i32)  [unwired: 3 in, 2 out]
        n150 = call "IMAQ ColorImageToArray"("Image"=w432) -> ("Image Pixels (U32)"=w433:u32[][])  [unwired: 3 in, 2 out]
        n151 = xnode "Read/Write Control"("FPGA VI Reference In"=w435, "StartOfImage"=w436) -> ()  [unwired: 1 in, 2 out]
        n152 = for {
          N: w434 -> [_]
          tunnel: w433 -> [w442] mode=indexing
          tunnel: [w442] -> w431 mode=concatenating
        }
        n153 = shared-variable "roboRIO-1256-FRC\\Shared Variable.lvlib\\sendNewPic"(w436) -> ()  [unwired: 1 in, 1 out]
        n154 = shared-variable-write(w430, w429, w431) -> (w428:refnum<k21>, w427:errorcluster)  [unwired: 1 in, 1 out]
      }
    }
    n155 = Or(x=w412, y="Stop") -> (x .or. y?=w420:bool)
  }
  n156 = Destroy Stream Endpoint(8:w32, 11:w31) -> (0:w25:errorcluster)
  n157 = Destroy Stream Endpoint(8:w43, 11:w44) -> (0:w26:errorcluster)
  n158 = Destroy Stream Endpoint(8:w46, 11:w45) -> (0:w27:errorcluster)
  n159 = Destroy Stream Endpoint(8:w81, 11:w82) -> (0:w77:errorcluster)
  n160 = Destroy Stream Endpoint(8:w66, 11:w65) -> (0:w64:errorcluster)
  n161 = Destroy Stream Endpoint(8:w6, 11:w7) -> ()  [unwired: 1 out]
  n162 = Destroy Stream Endpoint(8:w62, 11:w63) -> (0:w24:errorcluster)
  n163 = stacked-sequence {
    tunnel: w137 -> [w443]
    tunnel: [w443] -> w109
    frame #0 {
      n164 = local write "Stop"(TRUE ("Stop")) -> ()
    }
  }
  n165 = Destroy Stream Endpoint(8:w1, 11:w2) -> ()  [unwired: 1 out]
  n166 = case shown="Error" w95 {
    selector: w95 -> [w445 w446]
    tunnel: [w445 w446] -> w80
    frame No Error {
    }
    frame Error {
      n167 = shared-variable "roboRIO-1256-FRC\\Shared Variable.lvlib\\Active"(FALSE ("Active?")) -> ()  [unwired: 1 in, 1 out]
    }
  }
  n168 = Destroy Stream Endpoint(8:w55, 11:w56) -> (0:w28:errorcluster)
  n169 = xnode "Close FPGA VI Reference"("FPGA VI Reference In"=w138, "error in"=w109) -> ("error out"=w136:errorcluster)
  n170 = Destroy Stream Endpoint(8:w80, 11:w94) -> (0:w78:errorcluster)
  n171 = stacked-sequence {
    tunnel: w110 -> [w448]
    tunnel: [w448] -> w107
    frame #0 {
      n172 = local write "Stop"(TRUE ("Stop")) -> ()
    }
  }
  n173 = Destroy Stream Endpoint(8:w84, 11:w85) -> (0:→"OriImage Err out":errorcluster)
  n174 = Merge Errors(w107, w109) -> (w108:errorcluster)
  n175 = Merge Errors(w78, w77, w64, w28, w27, w26, w25, w24) -> (→"error out 2":errorcluster)
  n176 = call <vilib>:"IMAQdx Stop Acquisition.vi"("error in"=w107, "Session In"=w120) -> ("error out"=w121:errorcluster, "Session Out"=w122:T2)  [unwired: 8 in]
  n177 = xnode "Close FPGA VI Reference"("FPGA VI Reference In"=w111, "error in"=w108) -> ("error out"=w139:errorcluster)
  n178 = call <vilib>:"IMAQdx Close Camera.vi"("error in"=w121, "Session In"=w122) -> ("error out"=w119:errorcluster)  [unwired: 9 in]
  n179 = call "IMAQ Dispose"("Image"=w140, "error in (no error)"=w139) -> ("error out"=w135:errorcluster)  [unwired: 4 in]
  n180 = Merge Errors(w119, w135, w136) -> (w115:errorcluster)
  n181 = xnode "Close FPGA VI Reference"("FPGA VI Reference In"=w14, "error in"=w115) -> ("error out"=w114:errorcluster)
  "Error Out" <- w114
  n182 = stacked-sequence {
    tunnel: w114 -> [_]
    frame #0 {
      n183 = local write "Stop"(FALSE ("Stop")) -> ()
    }
  }
  "Count" <- 0
